vi "JKISM Module AsyncCall.vi"() -> ()   [LabVIEW 2014]
uses:
  user.lib/_NEVSTOP/JKI State Machine ++/JKI-State-Machine-Plus.lvlib
panel:
  out "error out":errorcluster
  in  "DoSth: DoC(error)":bool
  in  "DoSth: DoB":bool
  in  "DoSth: DoA":bool
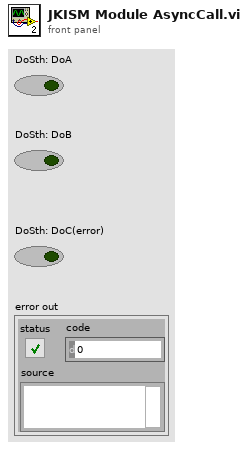
[diagram p1: front panel]
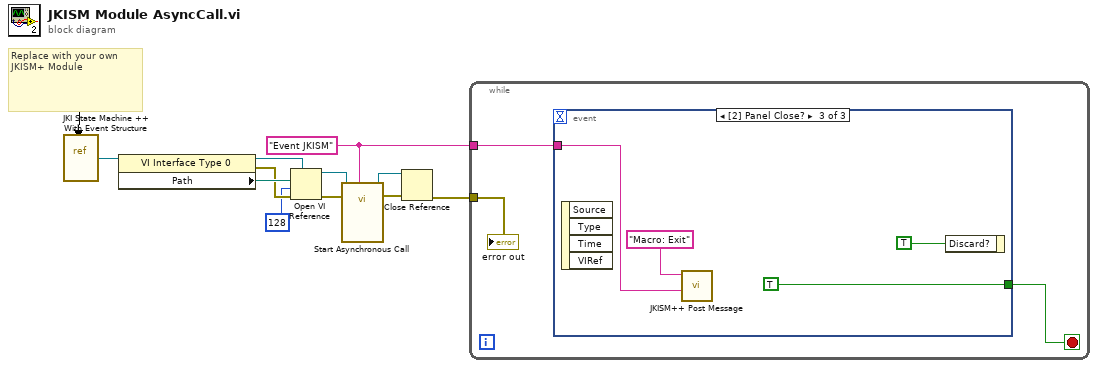
[diagram p0: block diagram]
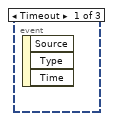
[diagram p2: hidden frame]
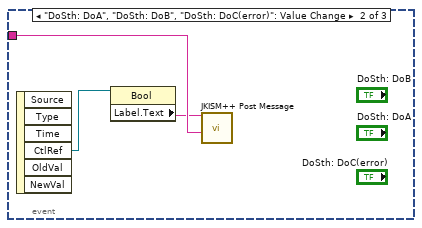
[diagram p3: hidden frame]
diagram:
  w1 = "Event JKISM" ("Name(\"\" to use uuid)")
  # "Replace with your own JKISM+ Module"
  n1 = vi-ref "JKI State Machine ++ With Event Structure.vi"() -> (w10:refnum<vi>)
  n2 = property class="VI Interface Type 0"(reference=w10) -> (reference out=w6:refnum<vi>, error out=w8:errorcluster, "Path"=w9:path)  [unwired: 1 in]
  n3 = Open VI Reference(type specifier VI Refnum (for type only)=w6, vi path=w9, options=128, error in (no error)=w8) -> (vi reference=w7:refnum<vi>, error out=w11:errorcluster)  [unwired: 2 in]
  n4 = call-by-ref "Start Asynchronous Call"(reference=w7, error in=w11, "Name(\"\" to use uuid)"=w1) -> (reference out=w4:refnum<vi>, error out=w5:errorcluster)  [unwired: 11 in]
  n5 = Close Reference(reference=w4, error in (no error)=w5) -> (error out=w3:errorcluster)
  n6 = while {
    tunnel: w1 -> [w13]
    tunnel: w3 -> [w12]
    stop <- w14 stop-if-true
    n7 = event shown="[2] Panel Close?" {
      selector: _ -> [_ _ _]
      dyn-events: _ -> [_ _ _]
      timeout: _ -> [_ _ _]
      tunnel: [_ _ TRUE ("Discard?")] -> w14
      tunnel: w13 -> [_ w17 w18]
      event Timeout {
        n8 = event-data() -> ()  [unwired: 1 in, 3 out]
      }
      event "DoSth: DoA", "DoSth: DoB", "DoSth: DoC(error)": Value Change {
        n9 = event-data() -> ("CtlRef"=w16:refnum<vi>)  [unwired: 1 in, 5 out]
        n10 = property class="Bool"(reference=w16) -> ("Label.Text"=w15:string)  [unwired: 1 in, 2 out]
        n11 = call "JKISM++ Post Message.vi"("Dest Module"=w17, "States"=w15) -> ()  [unwired: 9 in, 1 out]
      }
      event Panel Close? {
        n12 = event-data() -> ()  [unwired: 1 in, 4 out]
        n13 = call "JKISM++ Post Message.vi"("Dest Module"=w18, "States"="Macro: Exit") -> ()  [unwired: 9 in, 1 out]
        n14 = event-data("Discard?"=TRUE) -> ()  [unwired: 1 in, 1 out]
      }
    }
    "error out" <- w12
  }
